vi "MockDisplace.vi"(11 "MockDisplaceSettings":T1={"BufferUpdateFIFO"="MockDisplaceCommand", "DisplaceMeasurementMemory"="MockDisplaceMeasurements"}) -> ()   [LabVIEW 2016, in "FPGAMockDisplace.lvlib"]
uses:
  FPGAMockDisplace.lvlib
  DataTypes/MockDisplaceSettings.ctl
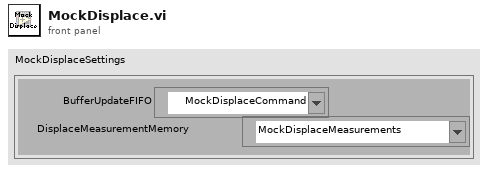
[diagram p1: front panel]
types:
  T1 = typedef "FPGAMockDisplace.lvlib/MockDisplaceSettings.ctl" = cluster{"BufferUpdateFIFO":refnum<k21>, "DisplaceMeasurementMemory":refnum<k21>}
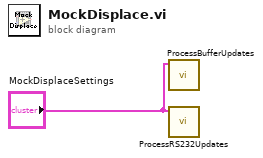
[diagram p0: block diagram]
diagram:
  n1 = call "ProcessBufferUpdates.vi"("MockDisplaceSettings"="MockDisplaceSettings") -> ()  [unwired: 11 in]
  n2 = call "ProcessRS232Updates.vi"("MockDisplaceSettings"="MockDisplaceSettings") -> ()  [unwired: 11 in]
